vi "GM emulator.vi"() -> ()   [LabVIEW 2014]
uses:
  <vilib>/Instr/_visa.llb/VISA Configure Serial Port (Instr).vi
panel:
  in  "baud rate (9600)":u32=19200
  in  "stop":bool
  out "Received string":string
  out "Cmd Rx.?":bool
  out "Bytes at Port":u32
  in  "VISA resource name":refnum<visa-resource-name>="COM6"
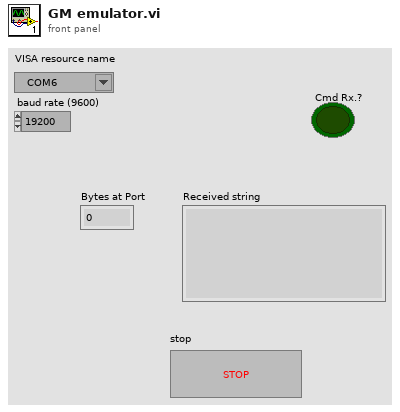
[diagram p1: front panel]
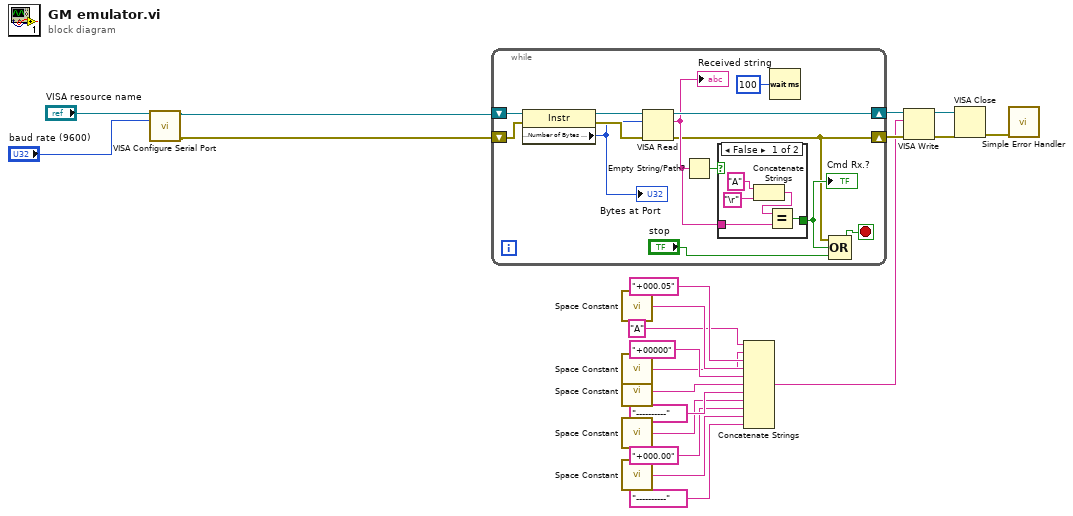
[diagram p0: block diagram]
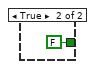
[diagram p2: hidden frame]
diagram:
  n1 = call-poly "VISA Configure Serial Port"("VISA resource name"="VISA resource name", "baud rate (9600)"="baud rate (9600)") -> ("VISA resource name out"=w2:refnum<visa-resource-name>, "error out"=w1:errorcluster)  [unwired: 12 in]
  n2 = while {
    shift-right: [w34] -> w20
    shift-left: w2 -> [w30]
    shift-right: [w23] -> w19
    shift-left: w1 -> [w31]
    stop <- w22 stop-if-true
    n3 = property class="Instr"(reference=w30, error in=w31) -> (reference out=w29:refnum<visa-resource-name>, error out=w28:errorcluster, "Serial Settings:Number of Bytes at Serial Port"=w27:u32)
    "Bytes at Port" <- w27
    n4 = VISA Read(VISA resource name=w29, byte count=w27, error in (no error)=w28) -> (VISA resource name out=w34:refnum<visa-resource-name>, read buffer=w32:string, error out=w23:errorcluster)  [unwired: 1 out]
    "Received string" <- w32
    n5 = Empty String/Path?(string/path=w32) -> (empty?=w33:bool)
    n6 = case shown="False" w33 {
      tunnel: [w39 FALSE] -> w24
      tunnel: w32 -> [w38 _]
      frame False {
        n7 = Concatenate Strings("A", "\r") -> (w35:string)
        n8 = Equal?(x=w35, y=w38) -> (x = y?=w39:bool)
      }
      frame True {
      }
    }
    "Cmd Rx.?" <- w24
    n9 = Wait (ms)(milliseconds to wait=u32 100) -> ()  [unwired: 1 out]
    n10 = Compound Arithmetic op=OR(w23, w24, "stop") -> (w22:bool)
  }
  n11 = call <vilib>:"Space Constant.vi"() -> ("String"=w11:string)
  n12 = call <vilib>:"Space Constant.vi"() -> ("String"=w9:string)
  n13 = call <vilib>:"Space Constant.vi"() -> ("String"=w17:string)
  n14 = call <vilib>:"Space Constant.vi"() -> ("String"=w15:string)
  n15 = call <vilib>:"Space Constant.vi"() -> ("String"=w13:string)
  n16 = Concatenate Strings("A", w9, "+000.05", w11, "+00000", w17, "----------", w15, "+000.00", w13, "----------") -> (w7:string)
  n17 = VISA Write(VISA resource name=w20, write buffer=w7, error in (no error)=w19) -> (VISA resource name out=w5:refnum<visa-resource-name>, error out=w6:errorcluster)  [unwired: 1 out]
  n18 = VISA Close(VISA resource name=w5, error in (no error)=w6) -> (error out=w4:errorcluster)
  n19 = call <vilib>:"Simple Error Handler.vi"("error in (no error)"=w4) -> ()  [unwired: 4 in, 5 out]
